vi "while loop.vi"() -> (3 "Numeric":i32)   [LabVIEW 2016]
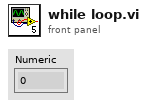
[diagram p1: front panel]
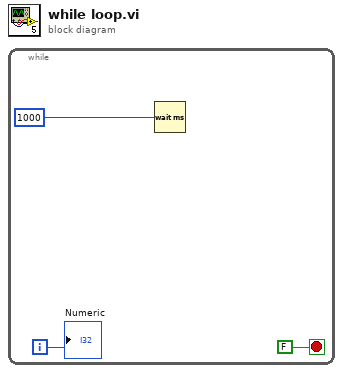
[diagram p0: block diagram]
diagram:
  n1 = while {
    i -> [w3]
    stop <- FALSE stop-if-true
    n2 = Wait (ms)(milliseconds to wait=u32 1000) -> ()  [unwired: 1 out]
    "Numeric" <- w3
  }
